vi "IDD Test_KGD.vi"(6 "script name":string="IDD", 8 "error in (no error)":errorcluster, 9 "Publishable IDs":string[](array[string])=["IDD_LowPower", "IDD_DVC_Cmin", "IDD_DVC_Cmax"], 10 "Pins":string[](array[string])=["VDD"], 11 "Semiconductor Module Context":T1) -> (0 "error out":errorcluster)   [LabVIEW 2013]
uses:
  <vilib>/NI_TestStand_SemiconductorModule/NI_TestStand_Semiconductor_Module.lvlibp/PinMap/General/SemiconductorModuleContext.ctl
  <instrlib>/niHSDIO/niHSDIO.llb/niHSDIO_ctl Trigger Script - trigID Values (Ring).ctl
  <vilib>/NI_TestStand_SemiconductorModule/NI_TestStand_Semiconductor_Module.lvlibp/PinMap/DC Power/PinsToNIDCPowerSessions.vi
  <vilib>/NI_TestStand_SemiconductorModule/NI_TestStand_Semiconductor_Module.lvlibp/PinMap/General/Publish/PublishDataDouble2D.vi
  <vilib>/NI_TestStand_SemiconductorModule/NI_TestStand_Semiconductor_Module.lvlibp
panel:
  out "current measurements":dbl[][](array[numeric])
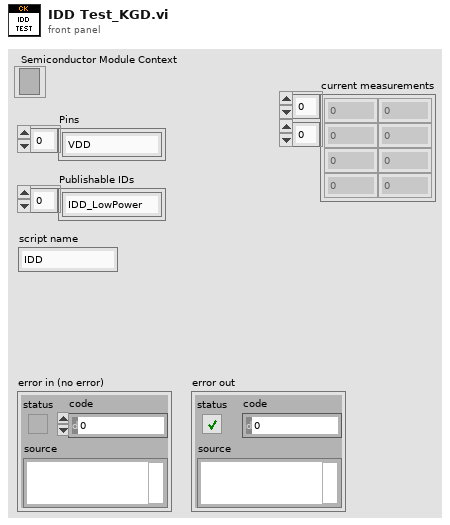
[diagram p1: front panel]
types:
  T1 = typedef "NI_TestStand_Semiconductor_Module.lvlibp/SemiconductorModuleContext.ctl" = refnum<k7>
  T2 = typedef "niHSDIO_ctl Trigger Script - trigID Values (Ring).ctl" = string
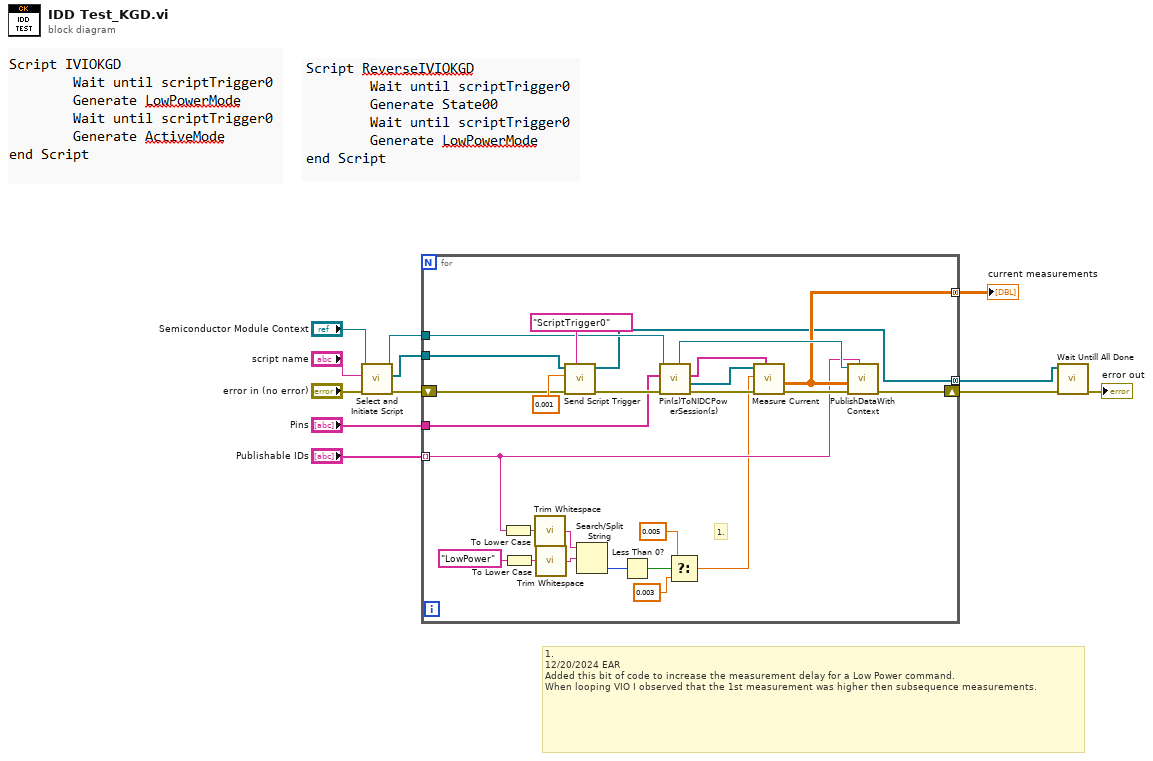
[diagram p0: block diagram]
diagram:
  # "1.\n12/20/2024 EAR\nAdded this bit of code to increase the measurement delay for a Low Power command. \nWhen looping VIO I observed that the 1st measurement was higher then subsequence measurements."
  n1 = call "Select and Initiate Script.vi"("error in (no error)"="error in (no error)", "script name"="script name", "Semiconductor Module Context"="Semiconductor Module Context") -> ("error out"=w3:errorcluster, "HSDIO GEN Sessions Out"=w7:refnum<k15>[], "Semiconductor Module Context Out"=w5:T1)  [unwired: 6 in]
  n2 = for {
    tunnel: "Pins" -> [w25]
    tunnel: w5 -> [w30]
    tunnel: w7 -> [w24]
    tunnel: "Publishable IDs" -> [w19] mode=indexing
    shift-right: [w33] -> w2
    shift-left: w3 -> [w26]
    tunnel: [w28] -> w8 mode=concatenating
    tunnel: [w27] -> w1 mode=concatenating
    # "1."
    n3 = To Lower Case(string=w19) -> (all lower case string=w23:string)
    n4 = To Lower Case(string="LowPower") -> (all lower case string=w22:string)
    n5 = call <vilib>:"Trim Whitespace.vi"("string"=w23) -> ("trimmed string"=w20:string)  [unwired: 1 in]
    n6 = call <vilib>:"Trim Whitespace.vi"("string"=w22) -> ("trimmed string"=w21:string)  [unwired: 1 in]
    n7 = call "Send Script Trigger.vi"("trigger id (script trigger 0)"=T2 "ScriptTrigger0", "error in (no error)"=w26, "Delay Time (s)"=0.001, "HSDIO Sessions In"=w24) -> ("error out"=w31:errorcluster, "HSDIO Sessions Out"=w27:refnum<k15>[])  [unwired: 6 in]
    n8 = Search/Split String(string=w20, search string/char (-)=w21) -> (offset of match=w17:i32)  [unwired: 1 in, 2 out]
    n9 = Less Than 0?(x=w17) -> (x < 0?=w16:bool)
    n10 = call-poly <vilib>:"Pin(s)ToNIDCPowerSession(s).vi"("error in (no error)"=w31, "Pins"=w25, "Semiconductor Module Context"=w30) -> ("error out"=w34:errorcluster, "Instrument Sessions"=w38:refnum<k15>[], "Channel Lists"=w36:string[], "Pin Query Context"=w35:refnum<class "MultiplePinMultipleSessionQueryContext.lvclass">)  [unwired: 4 in, 1 out]
    n11 = Select(t=0.005 ("Delay Time (s)"), s=w16, f=0.003 ("Delay Time (s)")) -> (s? t:f=w13:dbl)
    n12 = call "Measure Current.vi"("Channel Lists"=w36, "error in (no error)"=w34, "Delay Time (s)"=w13, "DCPower Sessions In"=w38) -> ("error out"=w37:errorcluster, "current measurements"=w28:dbl[][])  [unwired: 5 in, 1 out]
    n13 = call-poly <vilib>:"PublishDataWithContext.vi"("Published Data Id"=w19, "error in (no error)"=w37, "Data In"=w28, "Pin Query Context"=w35) -> ("error out"=w33:errorcluster)  [unwired: 6 in, 1 out]
  }
  "current measurements" <- w8
  n14 = call "Wait Untill All Done.vi"("error in (no error)"=w2, "HSDIO Sessions In"=w1) -> ("error out"=→"error out":errorcluster)  [unwired: 8 in, 1 out]
